vi "CheckFileRoot.vi"(10 "append letter":i8=65, 11 "File Name":string="none") -> (2 "append letter out":i8, 3 "FileNameOut":string)   [LabVIEW 2022 SP3]
uses:
  ScanningControl/Motion Controllers/-MotionRoutines/MotionGlobals.vi
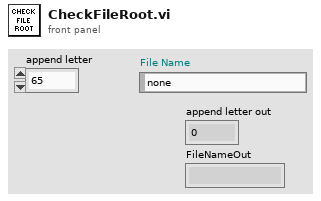
[diagram p1: front panel]
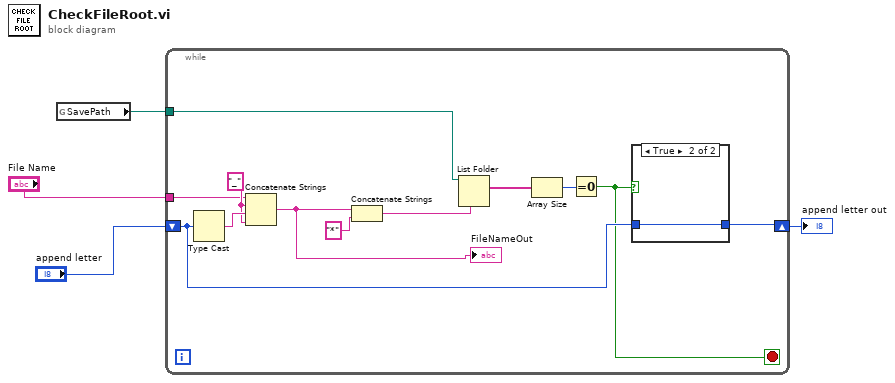
[diagram p0: block diagram]
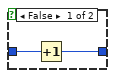
[diagram p2: hidden frame]
diagram:
  n1 = global read "MotionGlobals.vi" "SavePath"() -> (w2:path)
  n2 = while {
    tunnel: "File Name" -> [w11]
    tunnel: w2 -> [w10]
    shift-right: [w7] -> w1
    shift-left: "append letter" -> [w8]
    stop <- w6 stop-if-true
    w12 = "_" ("string")
    n3 = Type Cast(x=w8) -> (*(type *) &x=w13:string)  [unwired: 1 in]
    n4 = Concatenate Strings(w11, w12, w13, w12) -> (w5:string)
    "FileNameOut" <- w5
    n5 = Concatenate Strings(w5, "*") -> (w14:string)
    n6 = List Folder(path=w10, pattern=w14) -> (filenames=w15:string[])  [unwired: 1 in, 4 out]
    n7 = Array Size(array=w15) -> (size(s)=w9:i32)
    n8 = Equal To 0?(x=w9) -> (x = 0?=w6:bool)
    n9 = case shown="True" w6 {
      tunnel: w8 -> [w18 w19]
      tunnel: [w17 w19] -> w7
      frame False {
        n10 = Increment(x=w18) -> (x+1=w17:i8)
      }
      frame True {
      }
    }
  }
  "append letter out" <- w1
